vi "Autonomous Drive Delay.vi"(6 "Time":dbl, 8 "error in (no error)":errorcluster, 9 "Y":dbl, 10 "X":dbl, 11 "RobotDriveDevRef in":T1) -> (0 "error out":errorcluster, 3 "RobotDriveDevRef out":T1)   [LabVIEW 2013]
uses:
  <vilib>/Rock Robotics/WPI/RobotDrive/WPI_RobotDriveDevRef.ctl
  <vilib>/Rock Robotics/WPI/MotorControl/WPI_MotorControlDeviceRef.ctl
  <vilib>/Rock Robotics/SystemInterfaces/Typedef/FPGA_TypedefDigitalModule.ctl
  <vilib>/Rock Robotics/SystemInterfaces/DIO/FPGA_DIOPWMChannel.ctl
  <vilib>/Rock Robotics/WPI/PWM/WPI_PWMDeadband.ctl
  <vilib>/Rock Robotics/WPI/CAN/Jaguar/SubVIs/WPI_CANJaguar_ControlMode.ctl
  <vilib>/Rock Robotics/WPI/PWM/WPI_PWMTransform_ConPane.ctl
  <vilib>/Rock Robotics/WPI/RobotDrive/WPI_RobotDriveArcadeDrive_Standard(NoSaturation).vi
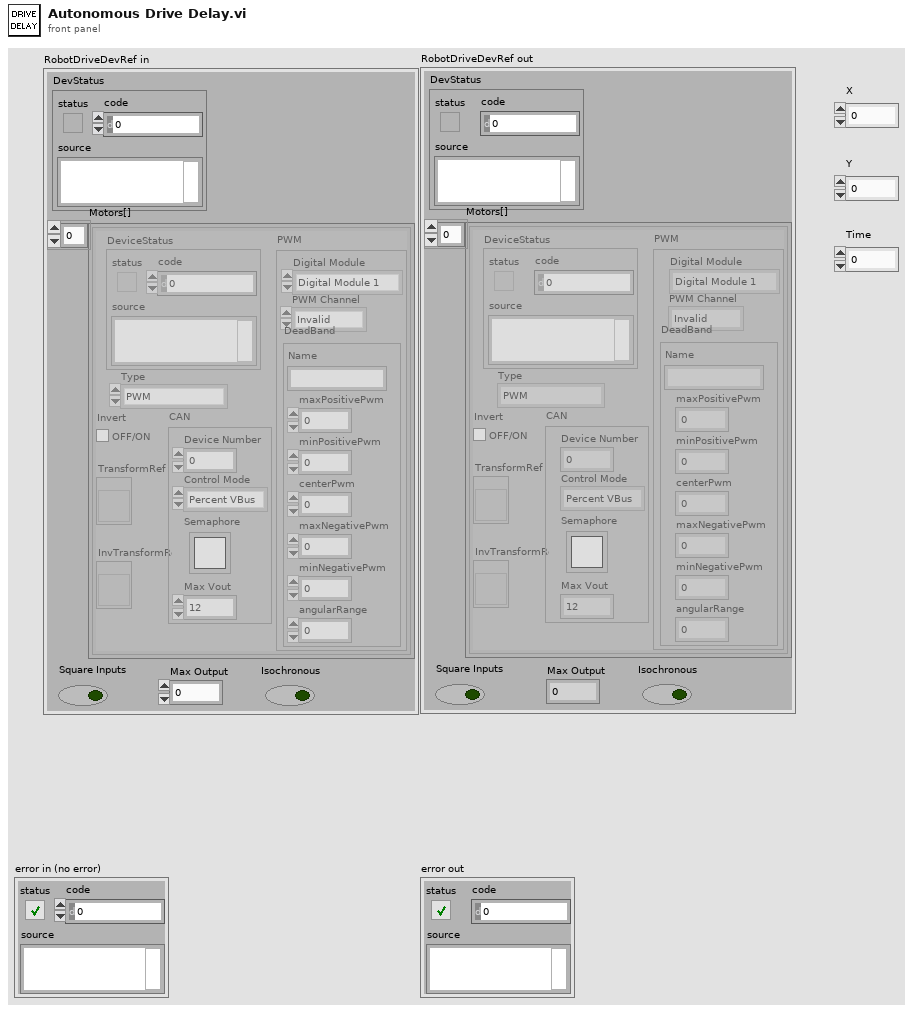
[diagram p1: front panel]
types:
  T1 = typedef "WPI_RobotDriveDevRef.ctl" = cluster{"DevStatus":errorcluster, "Motors[]":T2[], "Square Inputs":bool, "Max Output":dbl, "Isochronous":bool}
  T2 = typedef "WPI_MotorControlDeviceRef.ctl" = cluster{"DeviceStatus":errorcluster, "Type":enum16{"PWM", "CAN"}, "PWM":cluster{"Digital Module":T3, "PWM Channel":T4, "DeadBand":T5}, "CAN":cluster{"Device Number":u8, "Control Mode":T6, "Semaphore":T7, "Max Vout":dbl}, "Invert":bool, "TransformRef":T8, "InvTransformRef":T8}
  T3 = typedef "FPGA_TypedefDigitalModule.ctl" = enum16{"Digital Module 1", "Digital Module 2"}
  T4 = typedef "FPGA_DIOPWMChannel.ctl" = enum8{"PWM 1", "PWM 2", "PWM 3", "PWM 4", "PWM 5", "PWM 6", "PWM 7", "PWM 8", "PWM 9", "PWM 10", "Invalid"}
  T5 = typedef "WPI_PWMDeadband.ctl" = cluster{"Name":string, "maxPositivePwm":i32, "minPositivePwm":i32, "centerPwm":i32, "maxNegativePwm":i32, "minNegativePwm":i32, "angularRange":u16}
  T6 = typedef "WPI_CANJaguar_ControlMode.ctl" = enum8{"Percent VBus", "Current", "Speed", "Position", "Voltage"}
  T7 = typedef "Semaphore RefNum" = refnum<k1>
  T8 = typedef "WPI_PWMTransform_ConPane.ctl" = refnum<vi>
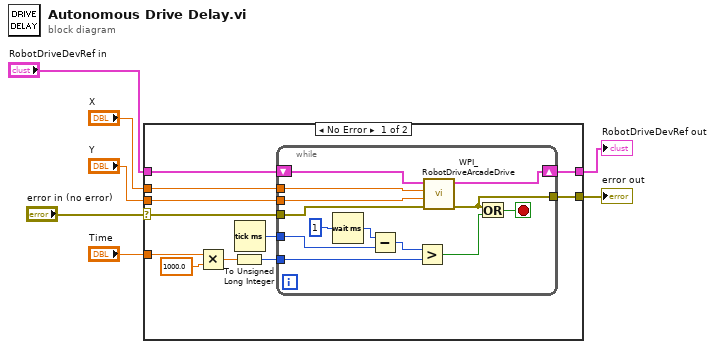
[diagram p0: block diagram]
diagram:
  n1 = case shown="No Error" "error in (no error)" {
    selector: "error in (no error)" -> [w13 w33]
    tunnel: "RobotDriveDevRef in" -> [w9 w32]
    tunnel: "Time" -> [w17 _]
    tunnel: [w12 w33] -> w5
    tunnel: [w8 w32] -> w4
    tunnel: "X" -> [w11 _]
    tunnel: "Y" -> [w10 _]
    frame No Error {
      n2 = Multiply(x=w17, y=1000.0) -> (x*y=w15:dbl)
      n3 = To Unsigned Long Integer(number=w15) -> (unsigned 32bit integer=w14:u32)
      n4 = Tick Count (ms)() -> (millisecond timer value=w18:u32)
      n5 = while {
        tunnel: w18 -> [w28]
        tunnel: w14 -> [w27]
        tunnel: w13 -> [w25]
        tunnel: [w23] -> w12
        tunnel: w11 -> [w22]
        tunnel: w10 -> [w21]
        shift-right: [w19] -> w8
        shift-left: w9 -> [w20]
        stop <- w24 stop-if-true
        n6 = Wait (ms)(milliseconds to wait=u32 1) -> (millisecond timer value=w29:u32)
        n7 = Subtract(x=w29, y=w28) -> (x-y=w30:u32)
        n8 = Greater?(x=w30, y=w27) -> (0:w26:bool)
        n9 = call-poly <vilib>:"WPI_RobotDriveArcadeDrive.vi"("error in (no error)"=w25, "Y axis value"=w21, "X axis value"=w22, "RobotDriveDevRef"=w20) -> ("error out"=w23:errorcluster, "RobotDriveDevRef"=w19:T1)  [unwired: 5 in, 1 out]
        n10 = Or(x=w23, y=w26) -> (x .or. y?=w24:bool)
      }
    }
    frame Error {
    }
  }
  "error out" <- w5
  "RobotDriveDevRef out" <- w4
